vi "DestroyPrivateEvents.vi"(8 "error in (no error)":errorcluster, 11 "DAQmx":refnum<class "DAQmx.lvclass">) -> (0 "error out":errorcluster, 3 "DAQmx out":refnum<class "DAQmx.lvclass">)   [LabVIEW 2019, in "DAQmx.lvclass"]
uses:
  DAQmx.lvclass
  <vilib>/JKI/JKI SMO/SMO/SMO.lvclass
panel:
  # "For instructions on how to use the JKI State Machine Objects, examples and video tutorials, visit:\nhttp://jki.net/state-machine-objects/\n\nJKI State Machine Objects™\nhttp://jki.net/state-machine-objects/\nCopyright (C) 2005-2015, JKI <info@jki.net>\nALL RIGHTS RESERVED"
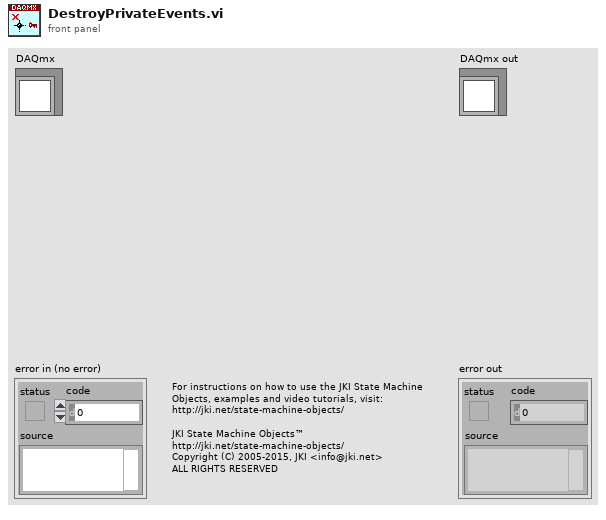
[diagram p1: front panel]
types:
  T1 = typedef "DAQmx.lvclass/PrivateEvents--Cluster.ctl" = cluster{"Message":refnum<user-event>, "AOconfig":refnum<user-event>, "AIconfig":refnum<user-event>, "Timing":refnum<user-event>}
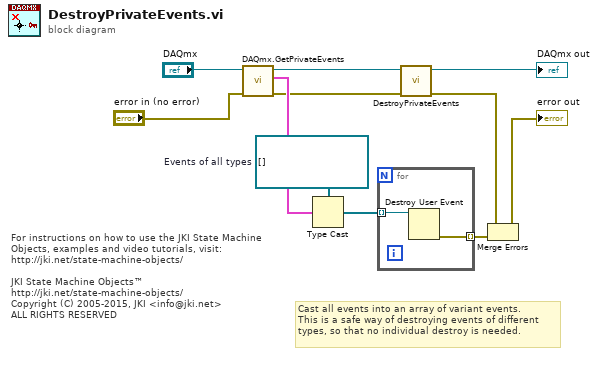
[diagram p0: block diagram]
diagram:
  w9 = refnum<user-event>[] []  # Events of all types
  # "For instructions on how to use the JKI State Machine Objects, examples and video tutorials, visit:\nhttp://jki.net/state-machine-objects/\n\nJKI State Machine Objects™\nhttp://jki.net/state-machine-objects/\nCopyright (C) 2005-2015, JKI <info@jki.net>\nALL RIGHTS RESERVED"
  # "Cast all events into an array of variant events.\nThis is a safe way of destroying events of different\ntypes, so that no individual destroy is needed."
  n1 = call "DAQmx.GetPrivateEvents.vi"("error in (no error)"="error in (no error)", "DAQmx"="DAQmx") -> ("error out"=w3:errorcluster, "DAQmx Private Events"=w5:T1, "DAQmx out"=w4:refnum<class "DAQmx.lvclass">)  [unwired: 7 in]
  n2 = Type Cast(type=w9, x=w5) -> (*(type *) &x=w10:refnum<user-event>[])
  n3 = for {
    tunnel: w10 -> [w13] mode=indexing
    tunnel: [w12] -> w8 mode=indexing
    n4 = Destroy User Event(user event=w13) -> (error out=w12:errorcluster)  [unwired: 1 in]
  }
  n5 = call-parent "DestroyPrivateEvents.vi"("error in (no error)"=w3, "SMO"=w4) -> ("error out"=w11:errorcluster, "SMO out"=→"DAQmx out":refnum<class "DAQmx.lvclass">)  [unwired: 8 in]
  n6 = Merge Errors(w11, w8) -> (→"error out":errorcluster)
